vi "TX_Mode Q Driver.vi"(0 "Q Name":string, 5 "State In":string, 7 "States s[]":string[](array[string]), 11 "error in (no error)":errorcluster, 13 "Q Operation":T1) -> (4 "State Out":string, 15 "error out":errorcluster)   [LabVIEW 2020, in "TX Speed.lvclass"]
uses:
  TX Speed.lvclass
  TypeDefs/TX_Mode Queue Operation Mode.ctl
  TX Speed.lvclass/TX Speed.ctl
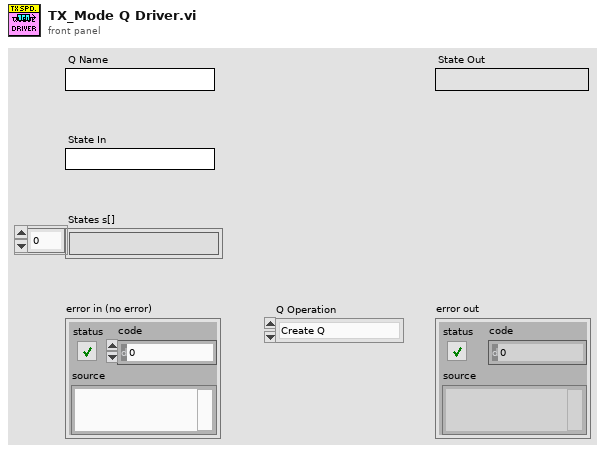
[diagram p1: front panel]
types:
  T1 = typedef "TX Speed.lvclass/TX_Mode Queue Operation Mode.ctl" = enum16{"Create Q", "Enqueue", "Enqueue N", "Enstack", "Dequeue", "Flush Q", "Close Q"}
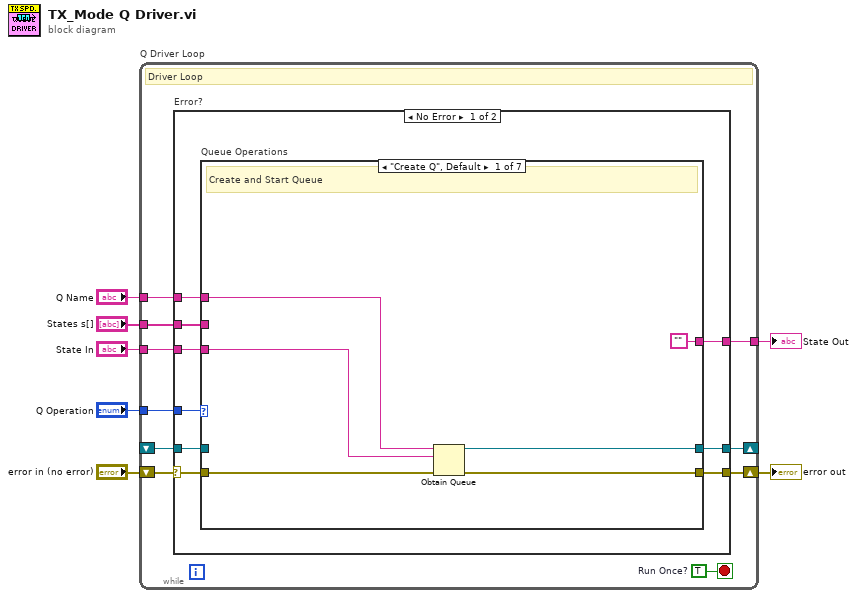
[diagram p0: block diagram]
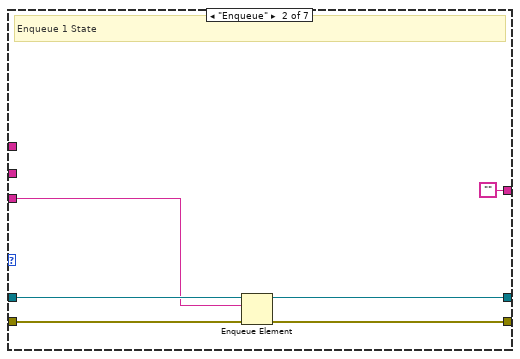
[diagram p2: hidden frame]
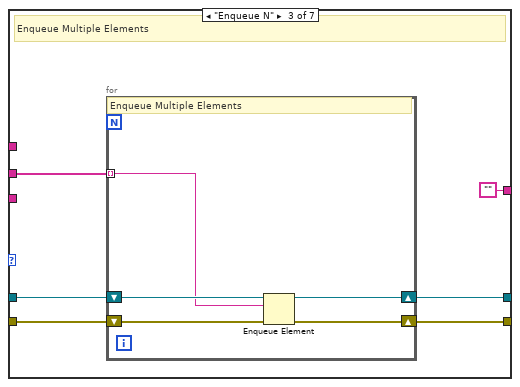
[diagram p3: hidden frame]
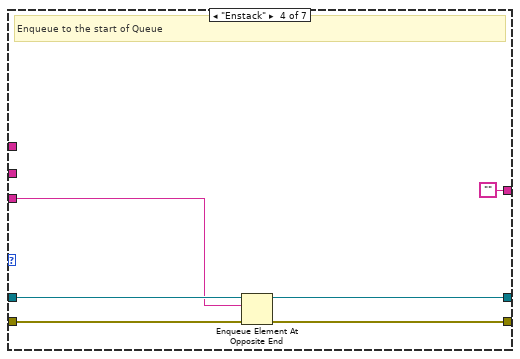
[diagram p4: hidden frame]
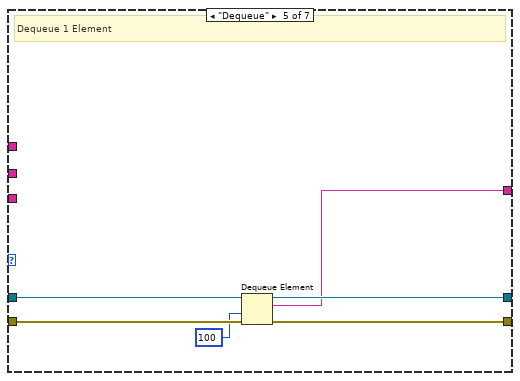
[diagram p5: hidden frame]
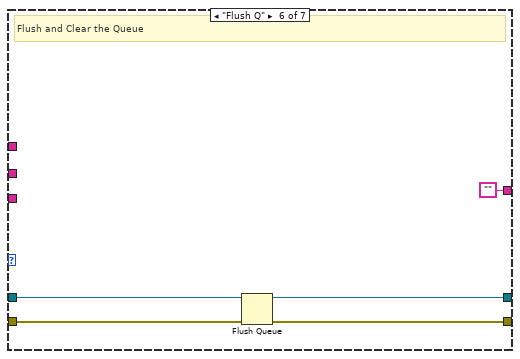
[diagram p6: hidden frame]
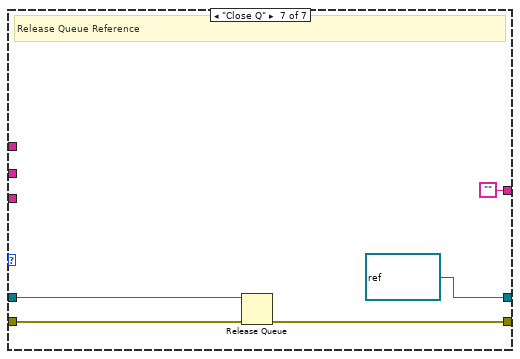
[diagram p7: hidden frame]
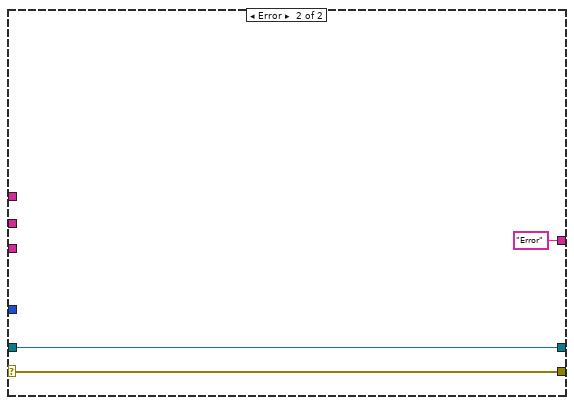
[diagram p8: hidden frame]
diagram:
  n1 = while "Q Driver Loop" {
    tunnel: "Q Operation" -> [w8]
    shift-right: [w15] -> _
    shift-left: _ -> [w14]
    tunnel: "States s[]" -> [w13]
    tunnel: "State In" -> [w12]
    tunnel: "Q Name" -> [w11]
    shift-right: [w16] -> w6
    shift-left: "error in (no error)" -> [w17]
    tunnel: [w10] -> w2
    stop <- w9 stop-if-true
    w9 = TRUE  # Run Once?
    # "Driver Loop"
    n2 = case "Error?" shown="No Error" w17 {
      selector: w17 -> [w25 w74]
      tunnel: [w26 w74] -> w16
      tunnel: w8 -> [w24 _]
      tunnel: [w23 w73] -> w15
      tunnel: w14 -> [w22 w73]
      tunnel: w13 -> [w21 _]
      tunnel: w12 -> [w20 _]
      tunnel: w11 -> [w19 _]
      tunnel: [w18 "Error"] -> w10
      frame No Error {
        n3 = case "Queue Operations" shown="\"Create Q\", Default" w24 {
          tunnel: [w31 w37 w44 w54 w60 w65 w70] -> w26
          tunnel: w25 -> [w32 w38 w43 w55 w61 w66 w71]
          tunnel: [w30 w35 w42 w51 w57 w63 refnum<queue> refnum ("queue out")] -> w23
          tunnel: w22 -> [_ w36 w41 w53 w59 w64 w69]
          tunnel: w21 -> [_ _ w40 _ _ _ _]
          tunnel: w20 -> [w27 w34 _ w52 _ _ _]
          tunnel: w19 -> [w29 _ _ _ _ _ _]
          tunnel: ["" ("Empty String Constant") "" ("Empty String Constant") "" ("Empty String Constant") "" ("Empty String Constant") w56 "" ("Empty String Constant") "" ("Empty String Constant")] -> w18
          frame "Create Q", Default {
            # "Create and Start Queue"
            n4 = Obtain Queue(name (unnamed)=w29, element data type=w27, error in (no error)=w32) -> (queue out=w30:refnum<queue>, error out=w31:errorcluster)  [unwired: 2 in, 1 out]
          }
          frame "Enqueue" {
            # "Enqueue 1 State"
            n5 = Enqueue Element(queue=w36, element=w34, error in (no error)=w38) -> (queue out=w35:refnum<queue>, error out=w37:errorcluster)  [unwired: 1 in, 1 out]
          }
          frame "Enqueue N" {
            # "Enqueue Multiple Elements"
            n6 = for {
              tunnel: w40 -> [w45] mode=indexing
              shift-right: [w48] -> w44
              shift-left: w43 -> [w49]
              shift-right: [w47] -> w42
              shift-left: w41 -> [w46]
              # "Enqueue Multiple Elements"
              n7 = Enqueue Element(queue=w46, element=w45, error in (no error)=w49) -> (queue out=w47:refnum<queue>, error out=w48:errorcluster)  [unwired: 1 in, 1 out]
            }
          }
          frame "Enstack" {
            # "Enqueue to the start of Queue"
            n8 = Enqueue Element At Opposite End(queue=w53, element=w52, error in (no error)=w55) -> (queue out=w51:refnum<queue>, error out=w54:errorcluster)  [unwired: 1 in, 1 out]
          }
          frame "Dequeue" {
            # "Dequeue 1 Element"
            n9 = Dequeue Element(queue=w59, timeout in ms (-1)=100, error in (no error)=w61) -> (queue out=w57:refnum<queue>, element=w56:string, error out=w60:errorcluster)  [unwired: 1 out]
          }
          frame "Flush Q" {
            # "Flush and Clear the Queue"
            n10 = Flush Queue(queue=w64, error in (no error)=w66) -> (queue out=w63:refnum<queue>, error out=w65:errorcluster)  [unwired: 1 out]
          }
          frame "Close Q" {
            # "Release Queue Reference"
            n11 = Release Queue(queue=w69, error in (no error)=w71) -> (error out=w70:errorcluster)  [unwired: 1 in, 2 out]
          }
        }
      }
      frame Error {
      }
    }
  }
  "error out" <- w6
  "State Out" <- w2
